vi "create stim logfile line (subVI).vi"(10 "step number":i32, 11 "relative seconds":dbl) -> (2 "string []":string[](array[string]))   [LabVIEW 2021]
uses:
  global-variables/global variables.vi
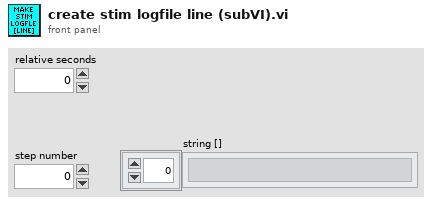
[diagram p1: front panel]
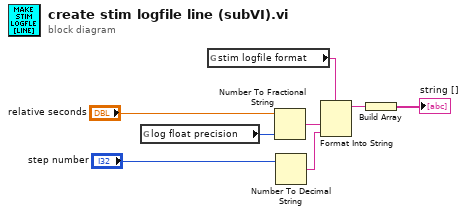
[diagram p0: block diagram]
diagram:
  n1 = global read "global variables.vi" "log float precision"() -> (w6:i16)
  n2 = global read "global variables.vi" "stim logfile format"() -> (w7:string)
  n3 = Number To Fractional String(number="relative seconds", precision (6)=w6) -> (F-format string=w2:string)  [unwired: 2 in]
  n4 = Number To Decimal String(number="step number") -> (decimal integer string=w5:string)  [unwired: 1 in]
  n5 = Format Into String(format string=w7, w2, w5) -> (resulting string=w3:string)  [unwired: 2 in, 1 out]
  n6 = Build Array(w3) -> (→"string []":string[])
